vi "Framework.Set Iteration.vi"(10 "iteration":u64, 11 "Framework in":refnum<class "Framework.lvclass">) -> (3 "Framework out":refnum<class "Framework.lvclass">)   [LabVIEW 2017, in "DSF Core.lvlib" / "Framework.lvclass"]
uses:
  Framework.lvclass
  Framework.lvclass/Framework.ctl
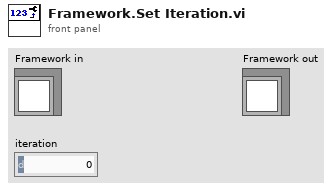
[diagram p1: front panel]
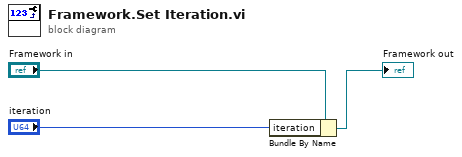
[diagram p0: block diagram]
diagram:
  n1 = Bundle By Name(cluster="Framework in", "iteration"="iteration") -> (→"Framework out":refnum<class "Framework.lvclass">)
